vi "receiver1.vi"() -> ()   [LabVIEW 2013]
uses:
  <vilib>/sound2/lvsound2.llb/Sound Data Format.ctl
  <instrlib>/niUSRP/niUSRP Fetch Rx Data (CDB WDT).vi
  <vilib>/Analysis/2dsp.llb/Rational Resample (single channel, DBL).vi
  <vilib>/sound2/lvsound2.llb/Sound Output Write (DBL Single).vi
  <vilib>/express/express analysis/Spectral/Block/exnSpectralBlock spectral measurements RMS poly.vi
  <vilib>/express/express analysis/Spectral/Block/exnSpectralBlock spectral measurements RMS WFM.vi
  <vilib>/express/express analysis/Spectral/XNode/ExpressSpectralMeasurementsBlockNode.xnode
  <vilib>/Analysis/NI_AALPro.lvlib
panel:
  out "XY Graph":cluster{dbl[], dbl[]}(graph)
  out "error out 2":errorcluster
  in  "sound format":T1={"sample rate (S/s)"=22050.0, "number of channels"=2, "bits per sample"=16}
  out "Spectrum (FFT)":cluster{"f0":dbl, "df":dbl, "magnitude":dbl[]}(graph)
  in  "stop":bool
  out "error out":errorcluster
  in  "number of samples":i64=1000
  out "coerced gain":dbl format="%#_6f"
  out "coerced carrier frequency":dbl=100000.0 format="%#_6p"
  out "coerced IQ rate":dbl=100000.0 format="%#_6p"
  in  "active antenna":string
  in  "gain":dbl format="%#_6f"
  in  "carrier frequency":dbl=100000.0 format="%#_6p"
  in  "IQ rate":dbl=100000.0 format="%#_6p"
  in  "device names":refnum<k15>
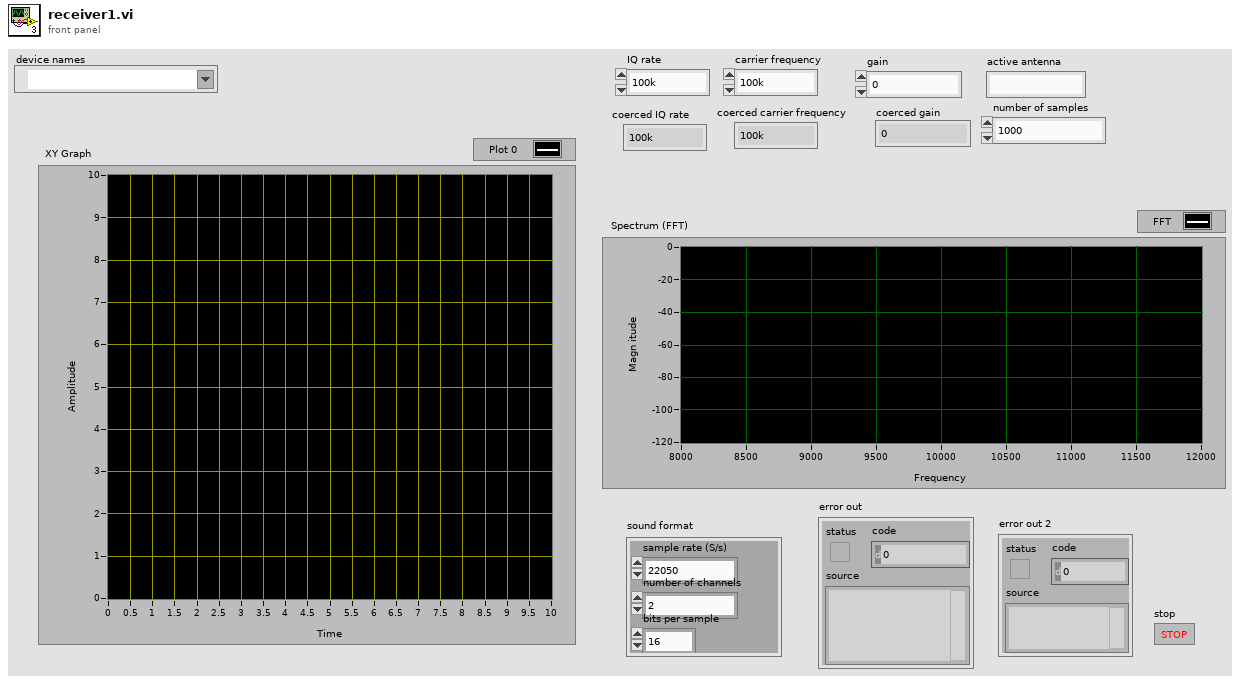
[diagram p1: front panel]
types:
  T1 = typedef "Sound Data Format.ctl" = cluster{"sample rate (S/s)":dbl, "number of channels":i32, "bits per sample":i32}
  T2 = typedef "Sound Output Task ID.ctl" = u32
  T3 = cluster{"averaging mode":u16, "weighting mode":u16, "number of averages":u32}
  T4 = cluster{"dB On (F)":bool, "unwrap phase (F)":bool, "convert to degree (F)":bool}
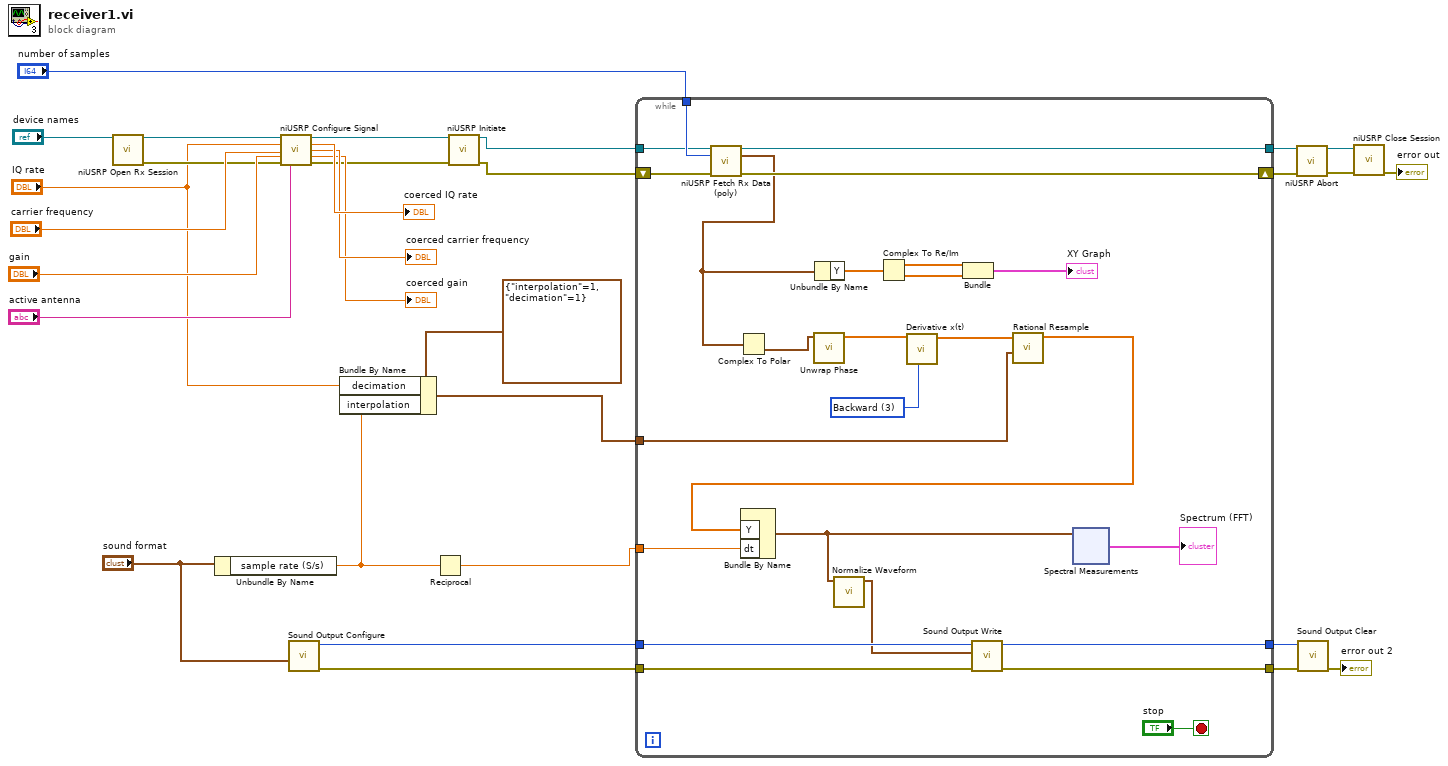
[diagram p0: block diagram]
diagram:
  n1 = call <instrlib>:"niUSRP Open Rx Session.vi"("device names"="device names") -> ("session handle out"=w12:refnum<k15>, "error out"=w13:errorcluster)  [unwired: 13 in]
  n2 = Unbundle By Name("sound format") -> ("sample rate (S/s)"=w3:dbl)
  n3 = call <instrlib>:"niUSRP Configure Signal.vi"("session handle"=w12, "IQ rate"="IQ rate", "carrier frequency"="carrier frequency", "gain"="gain", "error in (no error)"=w13, "active antenna"="active antenna") -> ("session handle out"=w24:refnum<k15>, "coerced IQ rate"=→"coerced IQ rate":dbl, "coerced carrier frequency"=→"coerced carrier frequency":dbl, "coerced gain"=→"coerced gain":dbl, "error out"=w23:errorcluster)  [unwired: 5 in]
  n4 = call <vilib>:"Sound Output Configure.vi"("sound format"="sound format") -> ("error out"=w8:errorcluster, "task ID"=w9:T2)  [unwired: 9 in]
  n5 = Bundle By Name(cluster=cluster{"interpolation":i32, "decimation":i32} {"interpolation"=1, "decimation"=1} ("input cluster"), "decimation"="IQ rate", "interpolation"=w3) -> (w2:cluster{"interpolation":i32, "decimation":i32})
  n6 = Reciprocal(x=w3) -> (1/x=w10:dbl)
  n7 = call <instrlib>:"niUSRP Initiate.vi"("session handle"=w24, "error in (no error)"=w23) -> ("session handle out"=w21:refnum<k15>, "error out"=w20:errorcluster)  [unwired: 12 in]
  n8 = while {
    tunnel: "number of samples" -> [w55]
    tunnel: w21 -> [w54]
    shift-right: [w51] -> w18
    shift-left: w20 -> [w53]
    tunnel: [w52] -> w19
    tunnel: w2 -> [w40]
    tunnel: w10 -> [w38]
    tunnel: w9 -> [w37]
    tunnel: w8 -> [w36]
    tunnel: [w35] -> w7
    tunnel: [w34] -> w6
    stop <- "stop" stop-if-true
    w42 = u16 3 items=["2nd Order Central", "4th Order Central", "Forward", "Backward"] ("method")
    n9 = call-poly <instrlib>:"niUSRP Fetch Rx Data (poly).vi"("session handle"=w54, "number of samples"=w55, "error in (no error)"=w53) -> ("session handle out"=w52:refnum<k15>, "data"=w45:waveform(cdb), "error out"=w51:errorcluster)  [unwired: 9 in, 1 out]
    n10 = Complex To Polar(r * e^(i*theta)=w45) -> (theta=w44:waveform(dbl))  [unwired: 1 out]
    n11 = call <vilib>:"Unwrap Phase.vi"("Phase"=w44) -> ("Unwrapped Phase"=w43:dbl[])  [unwired: 9 in, 1 out]
    n12 = Unbundle By Name(w45) -> ("Y"=w48:cdb[])
    n13 = Complex To Re/Im(x + iy=w48) -> (x=w47:dbl[], y=w46:dbl[])
    n14 = call <vilib>:"Derivative x(t).vi"("method"=w42, "X"=w43) -> ("dX/dt"=w41:dbl[])  [unwired: 8 in, 1 out]
    n15 = Bundle(w47, w46) -> (→"XY Graph":cluster{dbl[], dbl[]})  [unwired: 1 in]
    n16 = call-poly <vilib>:"Rational Resample.vi"("resample factor"=w40, "X"=w41) -> ("Y"=w39:dbl[])  [unwired: 7 in, 2 out]
    n17 = Bundle By Name("Y"=w39, "dt"=w38) -> (w32:waveform(dbl))  [unwired: 1 in]
    n18 = call <vilib>:"Normalize Waveform.vi"("waveform in"=w32) -> ("normalized waveform"=w31:waveform(dbl))  [unwired: 7 in, 3 out]
    n19 = call-poly <vilib>:"Sound Output Write.vi"("error in (no error)"=w36, "data"=w31, "task ID"=w37) -> ("error out"=w34:errorcluster, "task ID out"=w35:T2)  [unwired: 7 in]
    n20 = xnode "Spectral Measurements"("Signals"=w32) -> ("FFT - (RMS)"=→"Spectrum (FFT)":cluster{"f0":dbl, "df":dbl, "magnitude":dbl[]})  [unwired: 1 in, 2 out]
  }
  n21 = call <instrlib>:"niUSRP Abort.vi"("session handle"=w19, "error in (no error)"=w18) -> ("session handle out"=w16:refnum<k15>, "error out"=w17:errorcluster)  [unwired: 12 in]
  n22 = call <vilib>:"Sound Output Clear.vi"("error in (no error)"=w6, "task ID"=w7) -> ("error out"=→"error out 2":errorcluster)  [unwired: 9 in]
  n23 = call <instrlib>:"niUSRP Close Session.vi"("session handle"=w16, "error in (no error)"=w17) -> ("error out"=→"error out":errorcluster)  [unwired: 13 in]
